vi "LibSVM GridSearch.vi"(7 "libsvm":T3={"libsvm options"={"cache_size"=200.0, "eps"=0.001, "shrinking"=TRUE, "probability"=FALSE}, "libsvm weights"={"C"=1.0, "weight_label"=[], "weight"=[]}}, 8 "error in (no error)":errorcluster, 10 "Grid parameters":T7={"C start"=-5.0, "C end"=15.0, "C step"=2.0, "Gamma start"=-15.0, "Gamma end"=3.0, "Gamma step"=2.0, "K"=10, "random seed"=-1}, 11 "Problem":T5) -> (0 "error out":errorcluster, 1 "gamma":dbl[](array[numeric]), 2 "C":dbl[](array[numeric]), 3 "Confusion matrices":T4[](array[typedef]), 5 "Misclassification counts":i32[](array[numeric]))   [LabVIEW 2014]
doc: "Performs a gridsearch for the C-SVC (C) and RBF parameter (gamma). The cross-validation module supplied by libsvm is not used, as it would generate a different randomized split for each parameter value. This could skew the results for certain data sets (good splits / bad splits).\n\nThe grid search is performed using K-fold (default: 10) cross-validation."
uses:
  Controls/Grid parameters.ctl
  Wrapper API/Controls/svm_problem.ctl
  Wrapper API/Controls/svm_node.ctl
  Tools/Controls/Binary_ConfusionMatrix.ctl
  Controls/Options Training.ctl
  Controls/Parameters C_SVC.ctl
  Wrapper API/Controls/svm_kernel_type.ctl
  Controls/Kernel.ctl
  SubVIs/SVM Train C_SVC.vi
  <vilib>/Analysis/1siggen.llb/Ramp Pattern by Delta.vi
  <vilib>/gmath/interp.llb/Create Mesh Grid (2D) (x,y arrays).vi
  <userlib>/_OpenG.lib/array/array.llb/Delete Elements from 1D Array (DBL)__ogtk.vi
  <userlib>/_OpenG.lib/array/array.llb/Delete Elements from 1D Array (Variant)__ogtk.vi
  Wrapper API/svm_train.vi
  Wrapper API/svm_predict.vi
  <vilib>/Analysis/NI_AALBase.lvlib
  <vilib>/gmath/NI_Gmath.lvlib
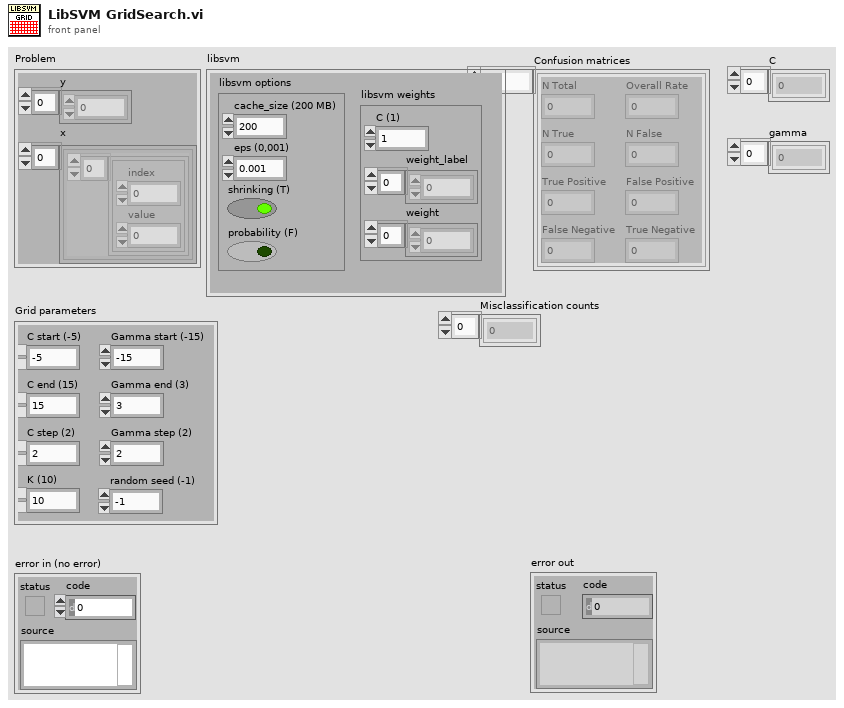
[diagram p1: front panel]
types:
  T1 = typedef "Options Training.ctl" = cluster{"cache_size":dbl, "eps":dbl, "shrinking":bool, "probability":bool}
  T2 = typedef "Parameters C_SVC.ctl" = cluster{"C":dbl, "weight_label":i32[], "weight":dbl[]}
  T3 = cluster{"libsvm options":T1, "libsvm weights":T2}
  T4 = typedef "Binary_ConfusionMatrix.ctl" = cluster{"N Total":u32, "N True":u32, "N False":u32, "Overall Rate":dbl, "True Positive":dbl, "False Positive":dbl, "False Negative":dbl, "True Negative":dbl}
  T5 = typedef "svm_problem.ctl" = cluster{"y":dbl[], "x":cluster{T6[]}[]}
  T6 = typedef "svm_node.ctl" = cluster{"index":i32, "value":dbl}
  T7 = typedef "Grid parameters.ctl" = cluster{"C start":dbl, "C end":dbl, "C step":dbl, "Gamma start":dbl, "Gamma end":dbl, "Gamma step":dbl, "K":i32, "random seed":i32}
  T8 = typedef "svm_kernel_type.ctl" = enum32{"LINEAR", "POLY", "RBF", "SIGMOID", "PRECOMPUTED"}
  T9 = typedef "Kernel.ctl" = cluster{"Type":T8, "Degree":i32, "Gamma":dbl, "Coef0":dbl}
  T10 = typedef "svm_model.ctl" = cluster{"param":T11, "nr_class":i32, "l":i32, "SV":cluster{"Array":T6[]}[], "sv_coef":dbl[][], "rho":dbl[], "probA":dbl[], "probB":dbl[], "sv_indices":i32[], "label":i32[], "nSV":i32[]}
  T11 = typedef "svm_parameter.ctl" = cluster{"svm_type":T12, "kernel_type":T8, "degree":i32, "gamma":dbl, "coef0":dbl, "cache_size":dbl, "eps":dbl, "C":dbl, "weight_label":i32[], "weight":dbl[], "nu":dbl, "p":dbl, "shrinking":bool, "probability":bool}
  T12 = typedef "svm_type.ctl" = enum32{"C_SVC", "NU_SVC", "ONE_CLASS", "EPSILON_SVR", "NU_SVR"}
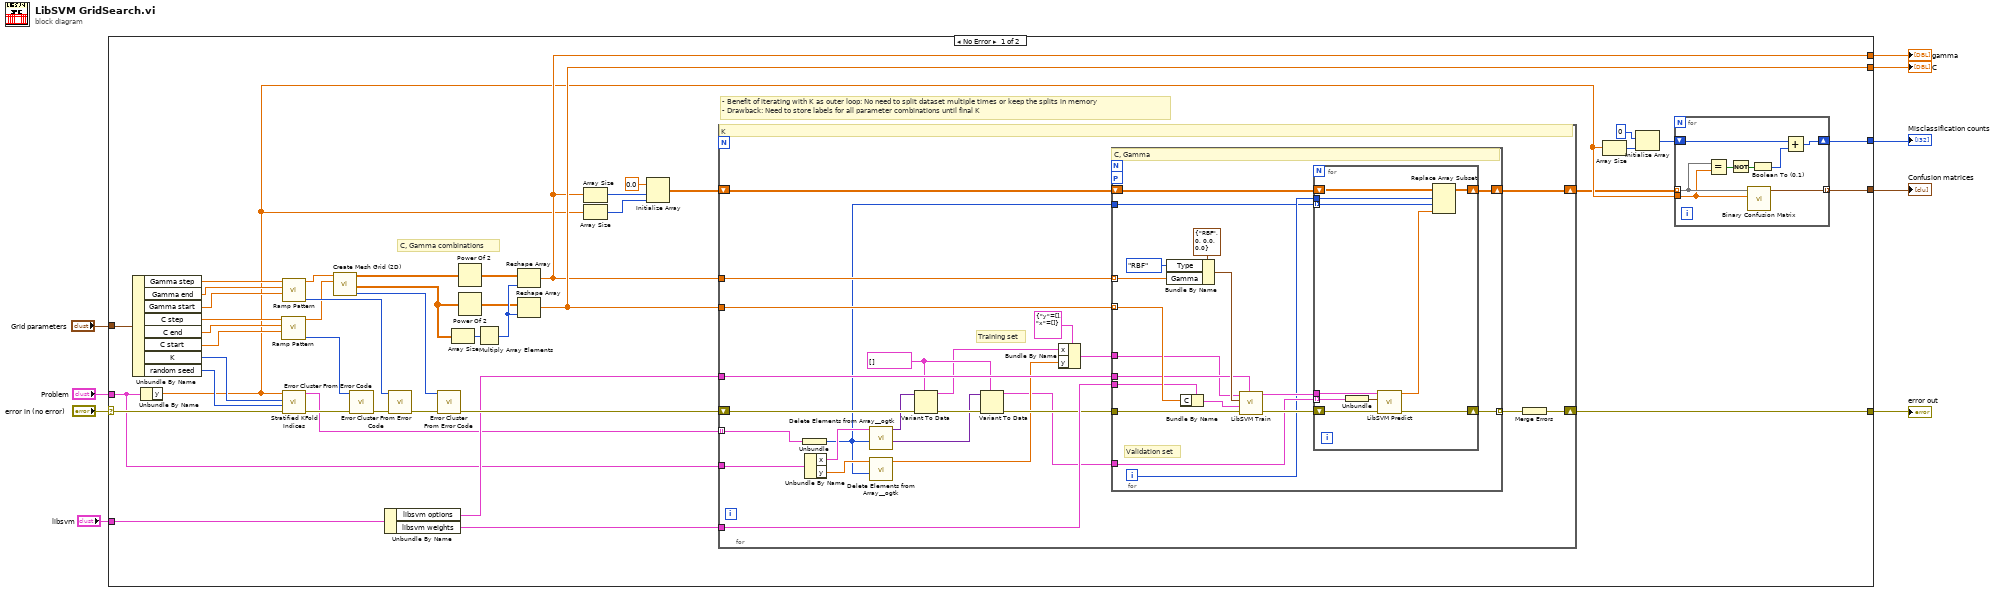
[diagram p0: block diagram]
diagram:
  n1 = case shown="No Error" "error in (no error)" {
    selector: "error in (no error)" -> [w33 w114]
    tunnel: [w11 w114] -> w9
    tunnel: "Problem" -> [w26 _]
    tunnel: "Grid parameters" -> [w53 _]
    tunnel: [w22 _] -> w5
    tunnel: [w27 _] -> w4
    tunnel: "libsvm" -> [w31 _]
    tunnel: [w12 _] -> w2
    tunnel: [w10 _] -> w1
    frame No Error {
      # "- Benefit of iterating with K as outer loop: No need to split dataset multiple times or keep the splits in memory\n- Drawback: Need to store labels for all parameter combinations until final K"
      # "C, Gamma combinations"
      n2 = Unbundle By Name(w53) -> ("Gamma step"=w52:dbl, "Gamma end"=w51:dbl, "Gamma start"=w50:dbl, "C step"=w49:dbl, "C end"=w48:dbl, "C start"=w47:dbl, "K"=w23:i32, "random seed"=w25:i32)
      n3 = Unbundle By Name(w26) -> ("y"=w17:dbl[])
      n4 = call-poly <vilib>:"Ramp Pattern.vi"("start"=w47, "end"=w48, "delta"=w49) -> ("error"=w45:i32, "Ramp Pattern"=w37:dbl[])  [unwired: 6 in, 1 out]
      n5 = call-poly <vilib>:"Ramp Pattern.vi"("start"=w50, "end"=w51, "delta"=w52) -> ("error"=w44:i32, "Ramp Pattern"=w38:dbl[])  [unwired: 6 in, 1 out]
      n6 = call "Stratified KFold Indices.vi"("error in (no error)"=w33, "seed"=w25, "Nr Folds"=w23, "Labels y"=w17) -> ("error out"=w32:errorcluster, "Stratified KFold indices"=w24:cluster{"elements":i32[]}[])  [unwired: 6 in]
      n7 = call-poly <vilib>:"Create Mesh Grid (2D).vi"("y domain"=w37, "x domain"=w38) -> ("error"=w42:i32, "Y"=w28:dbl[][], "X"=w36:dbl[][])  [unwired: 7 in]
      n8 = call <vilib>:"Error Cluster From Error Code.vi"("error in (no error)"=w32, "error code (0)"=w45) -> ("error out"=w46:errorcluster)  [unwired: 7 in]
      n9 = Unbundle By Name(w31) -> ("libsvm options"=w30:T1, "libsvm weights"=w29:T2)
      n10 = call <vilib>:"Error Cluster From Error Code.vi"("error in (no error)"=w46, "error code (0)"=w44) -> ("error out"=w43:errorcluster)  [unwired: 7 in]
      n11 = call <vilib>:"Error Cluster From Error Code.vi"("error in (no error)"=w43, "error code (0)"=w42) -> ("error out"=w39:errorcluster)  [unwired: 7 in]
      n12 = Array Size(array=w28) -> (size(s)=w41:i32[])
      n13 = Power Of 2(x=w36) -> (2^x=w35:dbl[][])
      n14 = Power Of 2(x=w28) -> (2^x=w34:dbl[][])
      n15 = Multiply Array Elements(1:w41) -> (0:w40:i32)
      n16 = Reshape Array(w35, w40) -> (w22:dbl[])
      n17 = Reshape Array(w34, w40) -> (w27:dbl[])
      n18 = Array Size(array=w22) -> (size(s)=w19:i32)
      n19 = Array Size(array=w17) -> (size(s)=w18:i32)
      n20 = Initialize Array(0.0 ("element"), w19, w18) -> (w20:dbl[][])
      n21 = for {
        tunnel: w22 -> [w85]
        tunnel: w27 -> [w84]
        tunnel: w29 -> [w83]
        tunnel: w30 -> [w82]
        tunnel: w26 -> [w81]
        tunnel: w24 -> [w62] mode=indexing
        shift-right: [w66] -> w13
        shift-left: w20 -> [w67]
        shift-right: [w63] -> w11
        shift-left: w39 -> [w79]
        w76 = cluster{T6[]}[] [] ("x")
        # "Training set"
        # "K"
        n22 = Unbundle(w62) -> ("elements"=w65:i32[])
        n23 = Unbundle By Name(w81) -> ("x"=w77:cluster{T6[]}[], "y"=w80:dbl[])
        n24 = call-poly <userlib>:"Delete Elements from Array__ogtk.vi"("indices"=w65, "array"=w77) -> ("deleted elements"=w75:variant[], "array w/ subset deleted"=w72:variant[])  [unwired: 8 in]
        n25 = call-poly <userlib>:"Delete Elements from Array__ogtk.vi"("indices"=w65, "array"=w80) -> ("array w/ subset deleted"=w70:dbl[])  [unwired: 8 in, 1 out]
        n26 = Variant To Data(error in=w79, type=w76, Variant=w72) -> (data=w71:cluster{T6[]}[], error out=w78:errorcluster)
        n27 = Variant To Data(error in=w78, type=w76, Variant=w75) -> (data=w68:cluster{T6[]}[], error out=w74:errorcluster)
        n28 = Bundle By Name(cluster=T5 {"y"=[], "x"=[]} ("Problem"), "x"=w71, "y"=w70) -> (w69:T5)
        n29 = for {
          tunnel: w85 -> [w101] mode=indexing
          tunnel: w84 -> [w100] mode=indexing
          tunnel: w83 -> [w99]
          tunnel: w82 -> [w92]
          workers-P: _ -> [_]
          tunnel: w69 -> [w91]
          tunnel: w68 -> [w90]
          shift-right: [w88] -> w66
          shift-left: w67 -> [w89]
          tunnel: w65 -> [w86]
          tunnel: w74 -> [w97]
          tunnel: [w93] -> w64 mode=indexing
          i -> [w87]
          # "Validation set"
          # "C, Gamma"
          n30 = Bundle By Name(cluster=T9 {"Type"=enum."RBF", "Degree"=0, "Gamma"=0.0, "Coef0"=0.0} ("Kernel"), "Type"=svm_kernel_type."RBF", "Gamma"=w101) -> (w96:T9)
          n31 = Bundle By Name(cluster=w99, "C"=w100) -> (w98:T2)
          n32 = call-poly "LibSVM Train.vi"("Options"=w92, "error in (no error)"=w97, "Param C_SVC"=w98, "Kernel"=w96, "Problem"=w91) -> ("error out"=w95:errorcluster, "Model"=w94:T10)  [unwired: 5 in]
          n33 = for {
            tunnel: w94 -> [w112]
            shift-right: [w109] -> w93
            shift-left: w95 -> [w110]
            tunnel: w90 -> [w113] mode=indexing
            shift-right: [w107] -> w88
            shift-left: w89 -> [w108]
            tunnel: w87 -> [w106]
            tunnel: w86 -> [w105] mode=indexing
            n34 = Unbundle(w113) -> (w111:T6[])
            n35 = call-poly "LibSVM Predict.vi"("error in (no error)"=w110, "X"=w111, "Model"=w112) -> ("error out"=w109:errorcluster, "Predicted label"=w104:dbl)  [unwired: 7 in]
            n36 = Replace Array Subset(array=w108, new element=w104, index (row)=w106, index (col)=w105) -> (w107:dbl[][])
          }
        }
        n37 = Merge Errors(w64) -> (w63:errorcluster)
      }
      n38 = Array Size(array=w17) -> (size(s)=w16:i32)
      n39 = Initialize Array(0, w16) -> (w14:i32[])
      n40 = for {
        tunnel: w13 -> [w61] mode=indexing
        tunnel: w17 -> [w60]
        shift-right: [w56] -> w10
        shift-left: w14 -> [w57]
        tunnel: [w54] -> w12 mode=indexing
        n41 = Equal?(x=w61, y=w60) -> (x = y?=w59:bool[])
        n42 = Not(x=w59) -> (.not. x?=w58:bool[])
        n43 = call "Binary Confusion Matrix.vi"("Actual Labels"=w60, "Predicted Labels"=w61) -> ("Binary Confusion Matrix"=w54:T4)  [unwired: 9 in]
        n44 = Boolean To (0,1)(Boolean=w58) -> (0, 1=w55:i16[])
        n45 = Add(x=w57, y=w55) -> (x+y=w56:i32[])
      }
    }
    frame Error {
    }
  }
  "error out" <- w9
  "Confusion matrices" <- w2
  "gamma" <- w5
  "C" <- w4
  "Misclassification counts" <- w1
